vi "Report_A170316-11.vi"(6 "文件重命名":bool, 7 "文件名称":string, 8 "错误输入（无错误）":errorcluster, 11 "布尔数组":bool[][](array[boolean])=[[TRUE]]) -> (0 "error out":errorcluster caption="错误输出")   [LabVIEW 2020]
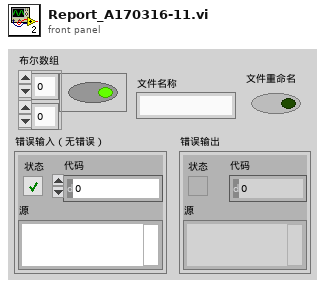
[diagram p1: front panel]
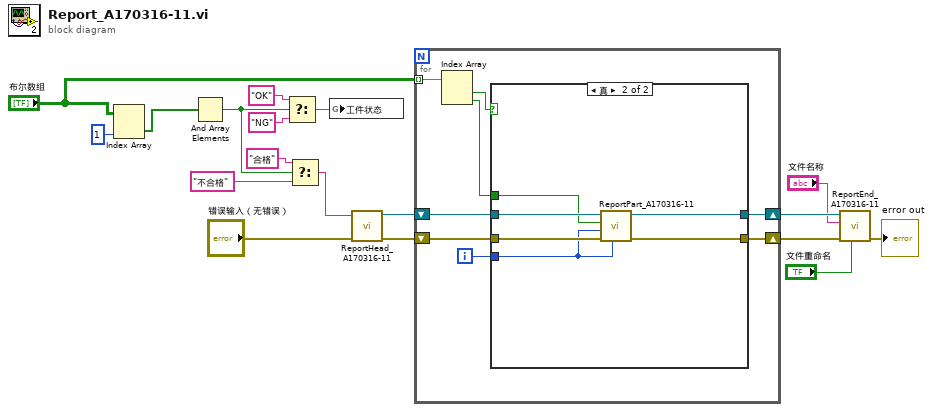
[diagram p0: block diagram]
diagram:
  n1 = Index Array(array="布尔数组", index (col)=1 ("禁用的索引 (列)")) -> (element=w2:bool[])  [unwired: 1 in]
  n2 = And Array Elements(Boolean array=w2) -> (logical AND=w5:bool)
  n3 = Select(t="OK", s=w5, f="NG") -> (s? t:f=w4:string)
  n4 = Select(t="合格", s=w5, f="不合格") -> (s? t:f=w8:string)
  n5 = global write "追溯全部变量.vi" "工件状态"(w4) -> ()
  n6 = call "ReportHead_A170316-11.vi"("error in (no error)"="错误输入（无错误）", "产品状态"=w8) -> ("error out"=w17:errorcluster, "report out"=w18:refnum<class "NI_report.lvclass">)  [unwired: 8 in]
  n7 = for {
    shift-right: [w24] -> w16
    shift-left: w18 -> [w26]
    shift-right: [w23] -> w15
    shift-left: w17 -> [w25]
    tunnel: "布尔数组" -> [w21] mode=indexing
    i -> [w22]
    n8 = Index Array(array=w21) -> (element #1=w20:bool, element #2=w19:bool)  [unwired: 2 in]
    n9 = case shown="真" w20 {
      tunnel: w26 -> [w27 w34]
      tunnel: w25 -> [w28 w33]
      tunnel: [w27 w32] -> w24
      tunnel: [w28 w31] -> w23
      tunnel: w22 -> [_ w29]
      tunnel: w19 -> [_ w30]
      frame False {
      }
      frame True {
        n10 = call "ReportPart_A170316-11.vi"("试验项目"=w29, "error in"=w33, "索引"=w29, "合格"=w30, "report in"=w34) -> ("error out"=w31:errorcluster, "report out"=w32:refnum<class "NI_report.lvclass">)  [unwired: 5 in]
      }
    }
  }
  n11 = call "ReportEnd_A170316-11.vi"("文件重命名"="文件重命名", "error in (no error)"=w15, "文件名称"="文件名称", "report in"=w16) -> ("error out"=→"error out":errorcluster)  [unwired: 7 in]
